vi "OSC converter.vi"(1 "1D OSC Configuration":T1(array[cluster])) -> (0 "2D OSC Configuration":T2(array[cluster]))   [LabVIEW 2013]
doc: "This subVI converts a 1D OSC configuration into a 2D OSC configuration."
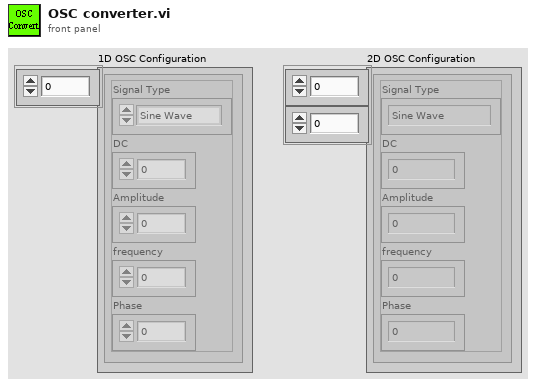
[diagram p1: front panel]
types:
  T1 = cluster{"Signal Type":enum16{"Sine Wave", "Triangle Wave", "Square Wave", "Sawtooth Wave"}, "DC":dbl, "Amplitude":dbl, "frequency":dbl, "Phase":dbl}[]
  T2 = cluster{"Signal Type":enum16{"Sine Wave", "Triangle Wave", "Square Wave", "Sawtooth Wave"}, "DC":dbl, "Amplitude":dbl, "frequency":dbl, "Phase":dbl}[][]
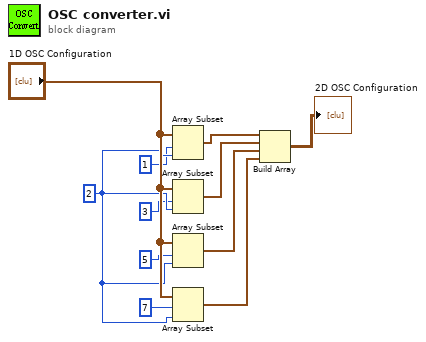
[diagram p0: block diagram]
diagram:
  w5 = 2
  n1 = Array Subset(array="1D OSC Configuration", index=1, length=w5) -> (w7:T1)
  n2 = Array Subset(array="1D OSC Configuration", index=3, length=w5) -> (w8:T1)
  n3 = Array Subset(array="1D OSC Configuration", index=5, length=w5) -> (w9:T1)
  n4 = Array Subset(array="1D OSC Configuration", index=7, length=w5) -> (w10:T1)
  n5 = Build Array(w7, w8, w9, w10) -> (→"2D OSC Configuration":T2)
